vi "GetAllBD-refs.vi"(8 "error in (no error)":errorcluster, 10 "Excluded objects":refnum<vi>[](array[refnum]), 11 "VI ref in":refnum<vi>) -> (0 "error out":errorcluster, 1 "All block diagram items (-filter)":refnum<vi>[](array[refnum]), 2 "Excluded objects out (dup)":refnum<vi>[](array[refnum]), 3 "VI ref out (dup)":refnum<vi>)   [LabVIEW 2017, in "ErrorStructureDrawer.lvlib"]
doc: "Get references to all Block Diagram objects, excluding any references listed in \"References to exclude\"."
uses:
  ErrorStructureDrawer.lvlib
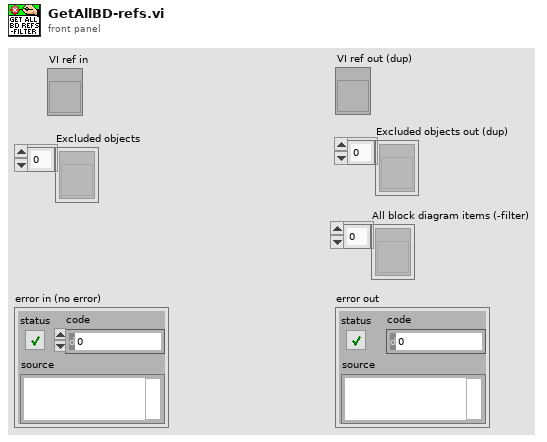
[diagram p1: front panel]
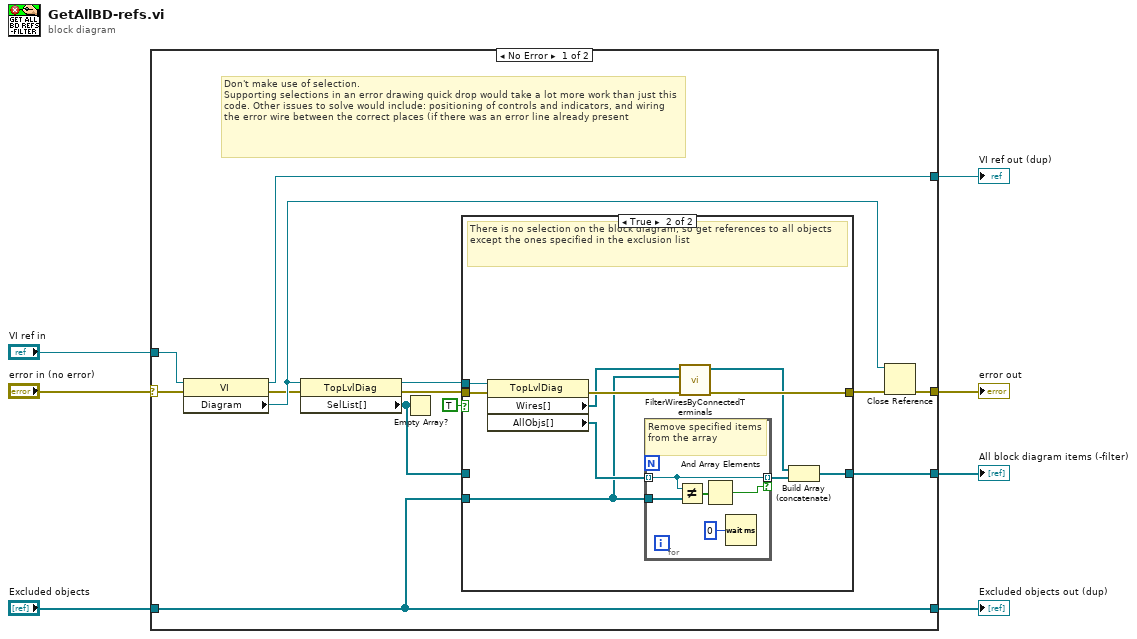
[diagram p0: block diagram]
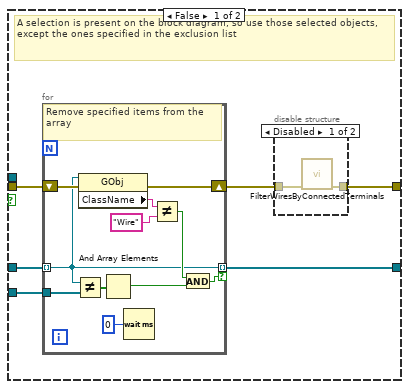
[diagram p2: hidden frame]
diagram:
  n1 = case shown="No Error" "error in (no error)" {
    selector: "error in (no error)" -> [w19 w58]
    tunnel: [w20 _] -> w7
    tunnel: [w18 w57] -> w6
    tunnel: [w16 w58] -> w5
    tunnel: "Excluded objects" -> [w14 w56]
    tunnel: "VI ref in" -> [w17 w57]
    tunnel: [w14 w56] -> w1
    frame No Error {
      # "Don't make use of selection.\nSupporting selections in an error drawing quick drop would take a lot more work than just this code. Other issues to solve would include: positioning of controls and indicators, and wiring the error wire between the correct places (if there was an error line already present"
      n2 = property class="VI"(reference=w17, error in=w19) -> (reference out=w18:refnum<vi>, error out=w11:errorcluster, "Diagram"=w13:refnum<vi>)
      n3 = property class="TopLvlDiag"(reference=w13, error in=w11) -> (reference out=w12:refnum<vi>, error out=w10:errorcluster, "SelList[]"=w9:refnum<vi>[])
      n4 = Empty Array?(array=w9) -> ()  [unwired: 1 out]
      n5 = case shown="True" TRUE {
        tunnel: [w23 w50] -> w20
        tunnel: w10 -> [w22 w48]
        tunnel: w12 -> [_ w47]
        tunnel: [w24 w45] -> w15
        tunnel: w14 -> [w26 w41]
        tunnel: w9 -> [w25 _]
        frame False {
          # "A selection is present on the block diagram, so use those selected objects, except the ones specified in the exclusion list"
          n6 = for {
            tunnel: w25 -> [w30] mode=indexing
            tunnel: w26 -> [w40]
            tunnel: [w30] -> w23 mode=indexing if=w36
            shift-right: [w31] -> w21
            shift-left: w22 -> [w32]
            # "Remove specified items from the array"
            n7 = Not Equal?(x=w30, y=w40) -> (x != y?=w39:bool[])
            n8 = property class="GObj"(reference=w30, error in=w32) -> (error out=w31:errorcluster, "ClassName"=w35:string)  [unwired: 1 out]
            n9 = And Array Elements(Boolean array=w39) -> (logical AND=w37:bool)
            n10 = Wait (ms)(milliseconds to wait=u32 0) -> ()  [unwired: 1 out]
            n11 = Not Equal?(x=w35, y="Wire") -> (x != y?=w33:bool)
            n12 = And(x=w33, y=w37) -> (x .and. y?=w36:bool)
          }
          n13 = disable-structure shown="Disabled" {
            disable-tunnel: w21 -> [w28 w29]
            disable-tunnel: [w27 w29] -> w24
            frame Disabled {
              n14 = call "FilterWiresByConnectedTerminals.vi"("error in (no error)"=w28) -> ("error out"=w27:errorcluster)  [unwired: 9 in, 1 out]
            }
            frame Enabled {
            }
          }
        }
        frame True {
          # "There is no selection on the block diagram, so get references to all objects except the ones specified in the exclusion list"
          n15 = property class="TopLvlDiag"(reference=w47, error in=w48) -> (error out=w46:errorcluster, "Wires[]"=w43:refnum<vi>[], "AllObjs[]"=w44:refnum<vi>[])  [unwired: 1 out]
          n16 = for {
            tunnel: w44 -> [w53] mode=indexing
            tunnel: w41 -> [w55]
            tunnel: [w53] -> w49 mode=indexing if=w52
            # "Remove specified items from the array"
            n17 = Not Equal?(x=w53, y=w55) -> (x != y?=w54:bool[])
            n18 = And Array Elements(Boolean array=w54) -> (logical AND=w52:bool)
            n19 = Wait (ms)(milliseconds to wait=u32 0) -> ()  [unwired: 1 out]
          }
          n20 = call "FilterWiresByConnectedTerminals.vi"("error in (no error)"=w46, "Excluded objects"=w41, "Wires in"=w43) -> ("error out"=w45:errorcluster, "Wires out (filtered)"=w42:refnum<vi>[])  [unwired: 7 in]
          n21 = Build Array (concatenate)(w42, w49) -> (w50:refnum<vi>[])
        }
      }
      n22 = Close Reference(reference=w13, error in (no error)=w15) -> (error out=w16:errorcluster)
    }
    frame Error {
    }
  }
  "All block diagram items (-filter)" <- w7
  "VI ref out (dup)" <- w6
  "error out" <- w5
  "Excluded objects out (dup)" <- w1
